vi "2D_template.vi"() -> ()   [LabVIEW 2014]
uses:
  support/Message Queue/Kapitza Message Queue.lvlib
  support/User Event - Stop/Kapitza User Event - Stop.lvlib
  support/Message Queue/Enqueue Message (Single).vi
  Classes/2D/IV/IV.lvclass
  Classes/2D/IV/data/IV_data.lvclass
  Classes/2D/IV/meas/IV_meas.lvclass
panel:
  in  "Additional Options_enum":enum32{"Page 1", "Page 2"}(tab)
  in  "Additional options":bool
  in  "Graphs":enum32{"IV", "dV/dI (I)"}(tab)
  out "IV":cluster{"X":dbl[], "Y":dbl[]}[](graph)
  out "dV/dI (I)":cluster{"X":dbl[], "Y":dbl[]}[](graph) caption="IV"
  out "Current Step":dbl
  out "dV/dI":dbl caption="dV/dI, Ohm"
  in  "File Path Control":path=path "C:/Users/Sergei/Documents"
  in  "Driver 1":path=path "C:/Users/Sergei/YandexDisk/Лаборатория/Projects/Kapitza_prealpha/Drivers/Simulator.vi" caption="Current source driver"
  in  "Driver 2":path=path "C:/Users/Sergei/YandexDisk/Лаборатория/Projects/Kapitza_prealpha/Drivers/Simulator.vi" caption="Voltmeter driver"
  in  "Address 2":refnum<visa-resource-name> caption="Voltmeter"
  in  "Address 1":refnum<visa-resource-name> caption="Current source"
  in  "Stop":bool
  in  "Sample Name":string
  in  "Max":dbl caption="Max current, uA"
  in  "Step":dbl caption="Current step, uA"
  in  "Init":dbl caption="Init current, uA"
  in  "x0,5 step":bool
  out "V":dbl caption="V, uV"
  out "I":dbl caption="I, uA"
  in  "x2 step":bool
  in  "Start":bool
  # "uA"
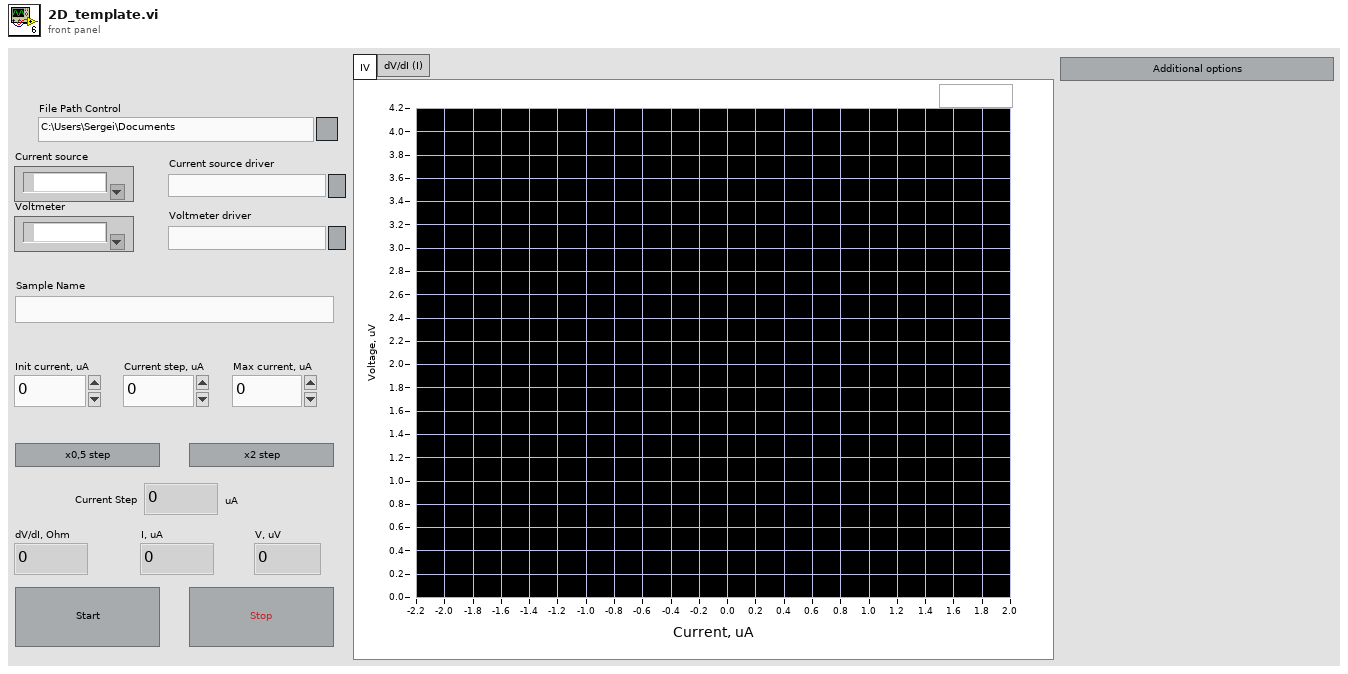
[diagram p1: front panel]
types:
  T1 = typedef "Kapitza Message Queue.lvlib/All Message Queues.ctl" = cluster{"UI":refnum<queue>}
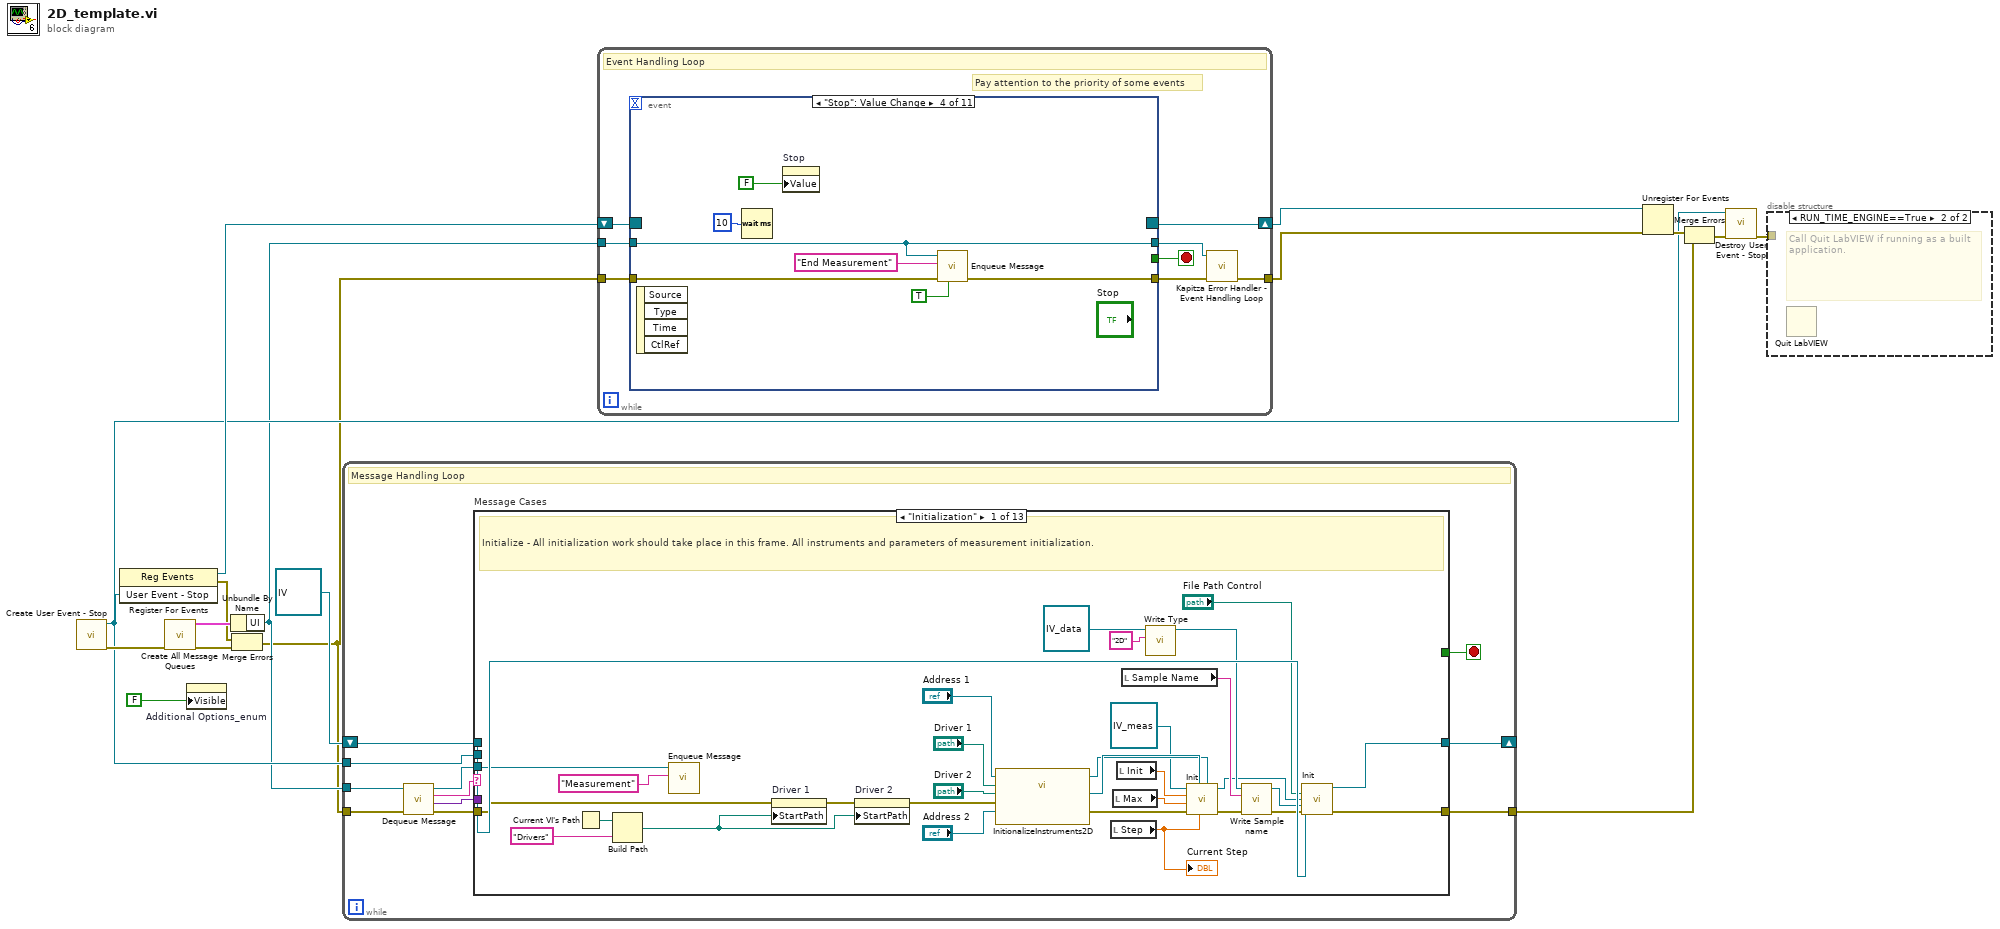
[diagram p0: block diagram]
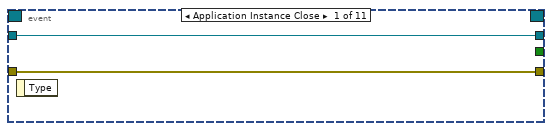
[diagram p3: hidden frame]
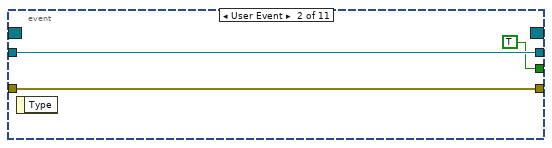
[diagram p4: hidden frame]
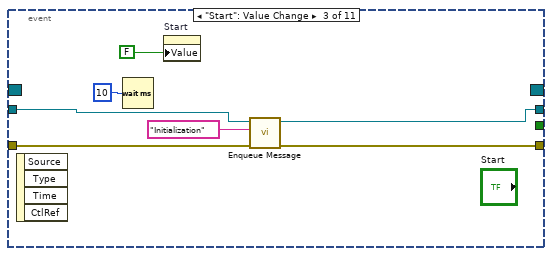
[diagram p5: hidden frame]
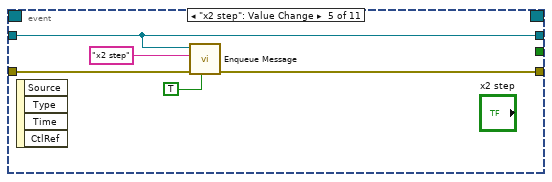
[diagram p6: hidden frame]
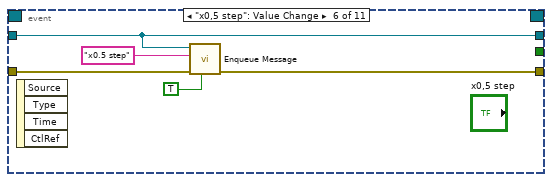
[diagram p7: hidden frame]
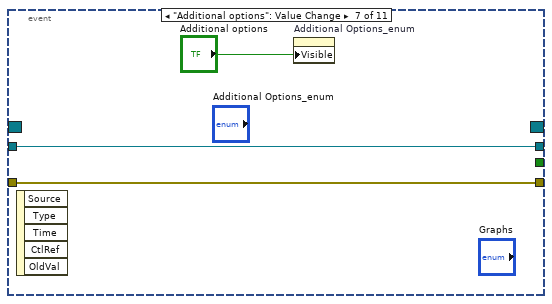
[diagram p8: hidden frame]
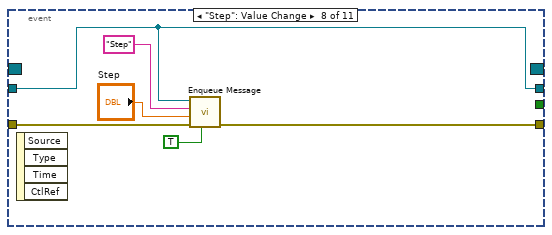
[diagram p9: hidden frame]
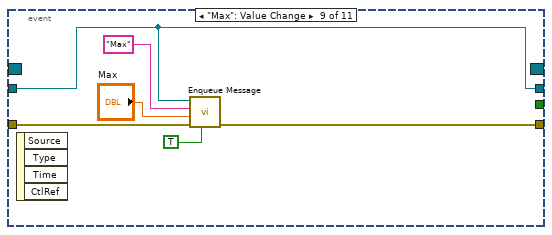
[diagram p10: hidden frame]
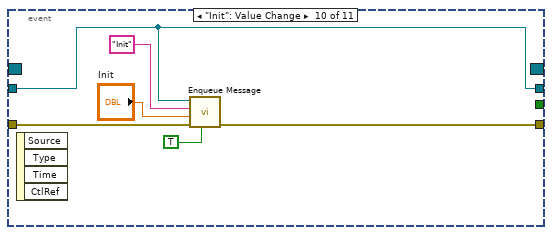
[diagram p11: hidden frame]
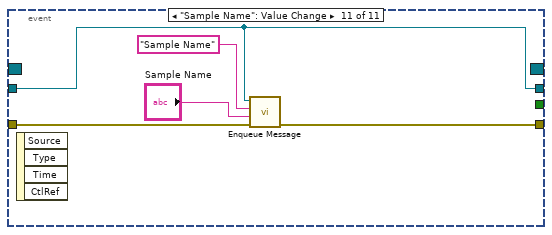
[diagram p12: hidden frame]
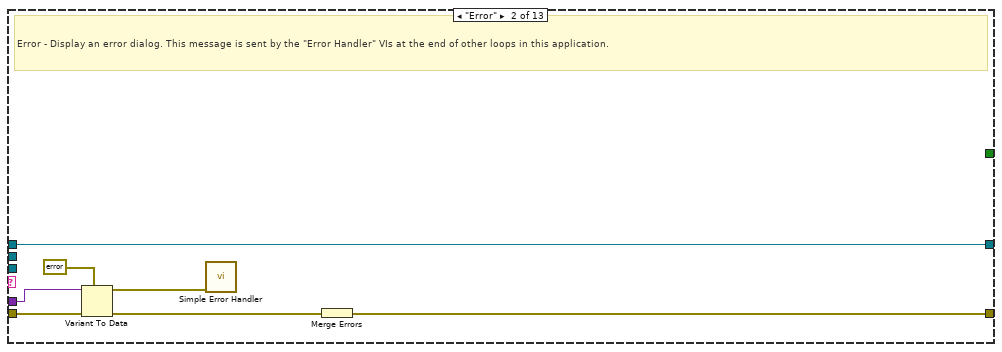
[diagram p13: hidden frame]
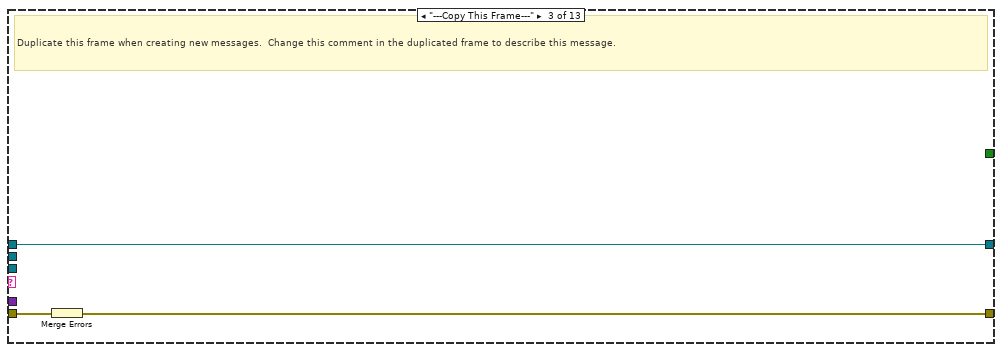
[diagram p14: hidden frame]
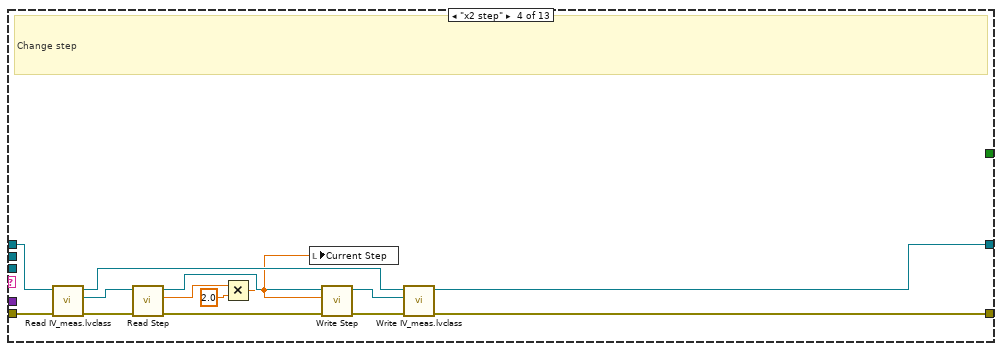
[diagram p15: hidden frame]
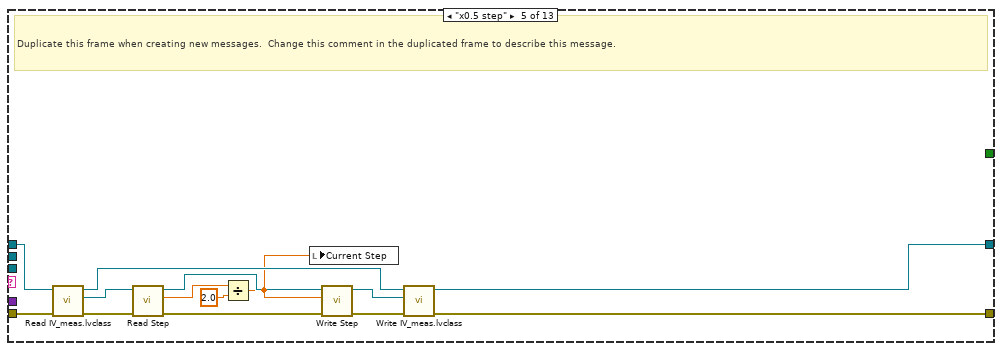
[diagram p16: hidden frame]
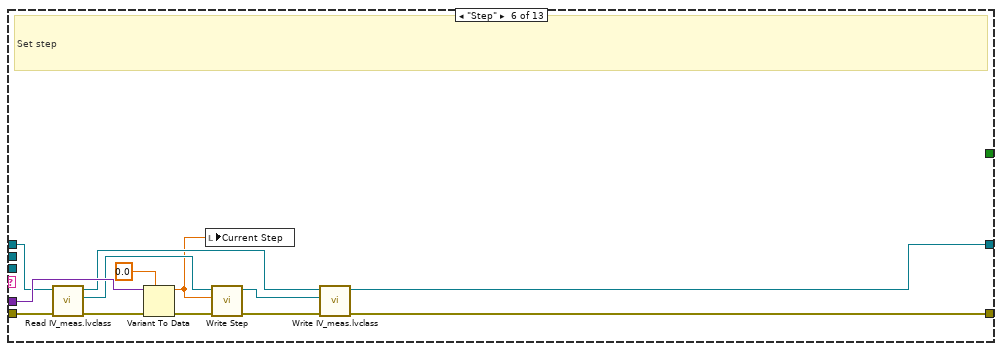
[diagram p17: hidden frame]
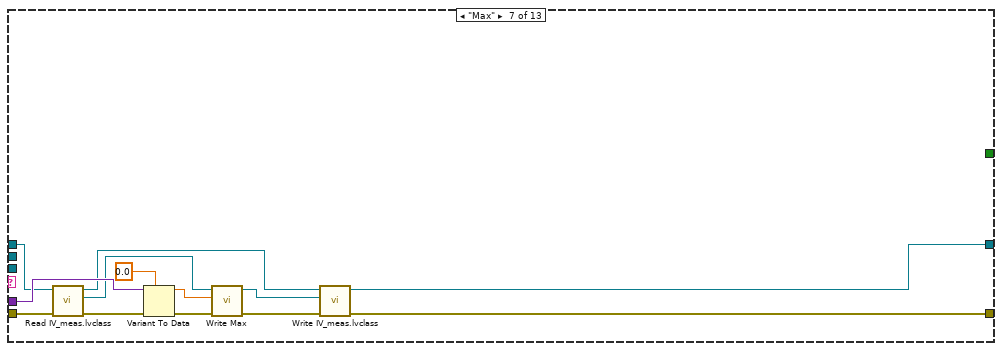
[diagram p18: hidden frame]
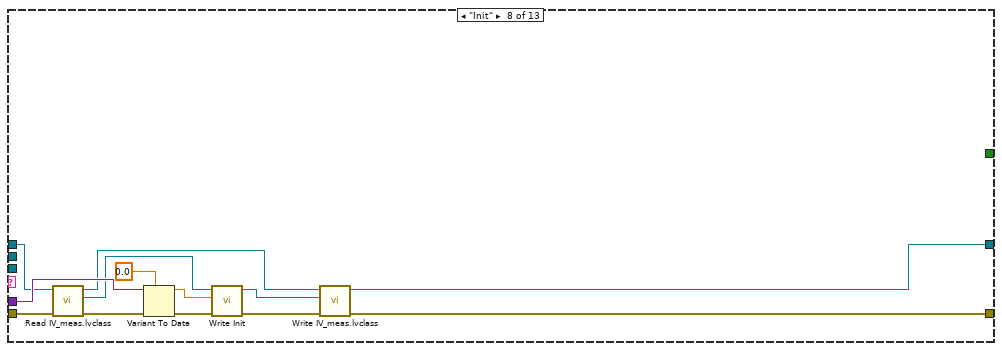
[diagram p19: hidden frame]
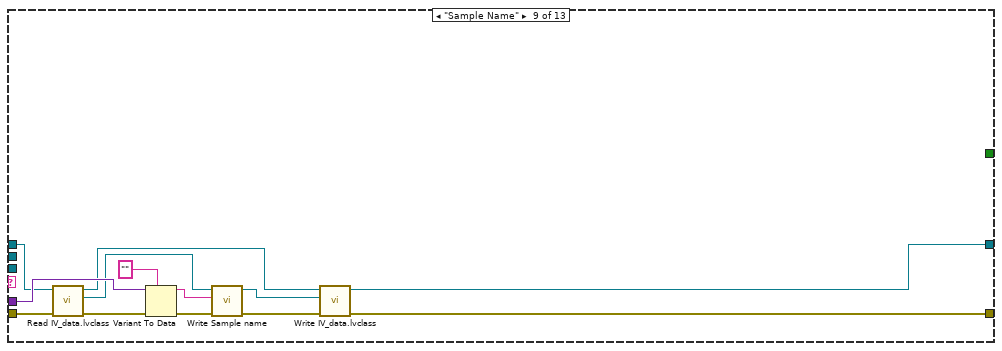
[diagram p20: hidden frame]
diagram:
  n1 = call "Create User Event - Stop.vi"() -> ("error out"=w14:errorcluster, "User Event - Stop"=w7:refnum<user-event>)  [unwired: 10 in]
  n2 = register-events(w7) -> (reference out=w8:refnum<event-registration>, error out=w6:errorcluster)  [unwired: 2 in]
  n3 = call "Create All Message Queues.vi"("error in (no error)"=w14) -> ("error out"=w4:errorcluster, "Message Queues out"=w16:T1)  [unwired: 9 in]
  n4 = property on="Additional Options_enum" class="TabCtl (strict)"("Visible"=FALSE) -> ()  [unwired: 2 in, 2 out]
  n5 = Unbundle By Name(w16) -> ("UI"=w5:refnum<queue>)
  n6 = Merge Errors(w6, w4) -> (w1:errorcluster)
  n7 = while {
    tunnel: w5 -> [w18]
    shift-right: [w26] -> _
    shift-left: refnum<class "IV.lvclass"> refnum ("IV.lvclass") -> [w27]
    tunnel: w7 -> [w24]
    tunnel: w1 -> [w23]
    tunnel: [w17] -> w15
    stop <- w25 stop-if-true
    # "Message Handling Loop"
    n8 = call "Dequeue Message.vi"("error in (no error)"=w23, "Message Queue"=w18) -> ("error out"=w22:errorcluster, "Message Data"=w20:variant, "Message"=w21:string, "dup Message Queue"=w19:refnum<queue>)  [unwired: 6 in]
    n9 = case "Message Cases" shown="\"Initialization\"" w21 {
      tunnel: w19 -> [w40 _ _ _ _ _ _ _ _ w158 w183 w195 _]
      tunnel: w22 -> [w45 w65 w68 w76 w84 w101 w115 w129 w141 w157 w177 w188 w196]
      tunnel: [w29 w59 w66 w75 w85 w103 w111 w131 w140 w155 w182 w191 w196] -> w17
      tunnel: w27 -> [w58 w64 w67 w77 w87 w107 w120 w130 w146 w159 w184 w194 w197]
      tunnel: [w30 w64 w67 w70 w86 w104 w110 w132 w139 w154 w170 w194 w197] -> w26
      tunnel: [_ _ _ _ _ _ _ _ _ _ _ TRUE _] -> w25
      tunnel: w20 -> [_ w63 _ _ _ w109 w122 w135 w148 _ _ w185 _]
      tunnel: w24 -> [_ _ _ _ _ _ _ _ _ _ _ w190 _]
      frame "Initialization" {
        # "Initialize - All initialization work should take place in this frame. All instruments and parameters of measurement initialization."
        n10 = Current VI's Path() -> (path=w47:path)
        n11 = Build Path(base path=w47, name or relative path="Drivers") -> (appended path=w43:path)
        n12 = call-poly "Enqueue Message.vi"("Message"="Measurement", "Message Queue"=w40) -> ()  [unwired: 8 in, 2 out]
        n13 = property on="Driver 1" class="Path"(error in=w45, "StartPath"=w43) -> (error out=w44:errorcluster)  [unwired: 1 in, 1 out]
        n14 = property on="Driver 2" class="Path"(error in=w44, "StartPath"=w43) -> (error out=w42:errorcluster)  [unwired: 1 in, 1 out]
        n15 = call "InitionalizeInstruments2D.vi"("Address in"="Address 2", "error in (no error)"=w42, "Driver in"="Driver 2", "Driver 1"="Driver 1", "VISA Refnum in"="Address 1") -> ("error out"=w50:errorcluster, "Instrument out 2"=w53:refnum<class "Instrument.lvclass">, "Instrument out"=w52:refnum<class "Instrument.lvclass">)  [unwired: 4 in]
        n16 = local read "Step"() -> (w28:dbl)
        "Current Step" <- w28
        n17 = local read "Max"() -> (w31:dbl)
        n18 = local read "Init"() -> (w32:dbl)
        n19 = local read "Sample Name"() -> (w51:string)
        n20 = call "Write Type.vi"("Type"="2D", "IV_data in"=refnum<class "IV_data.lvclass"> refnum ("IV_data.lvclass")) -> ("IV_data out"=w38:refnum<class "IV_data.lvclass">)  [unwired: 8 in, 1 out]
        n21 = call-dynamic "Init.vi"("Instrument.lvclass 2"=w52, "Step"=w28, "Instrument.lvclass"=w53, "error in (no error)"=w50, "Max"=w31, "Init"=w32, "Measurement1D in"=refnum<class "IV_meas.lvclass"> refnum ("IV_meas.lvclass")) -> ("error out"=w49:errorcluster, "Measurement1D out"=w34:refnum<class "IV_meas.lvclass">)  [unwired: 3 in]
        n22 = call "Write Sample name.vi"("error in (no error)"=w49, "Sample name"=w51, "IV_data in"=w38) -> ("error out"=w48:errorcluster, "IV_data out"=w33:refnum<class "IV_data.lvclass">)  [unwired: 7 in]
        n23 = call-dynamic "Init.vi"("IV in"=w58, "Path"="File Path Control", "IV_meas.lvclass"=w34, "IV_data.lvclass"=w33, "error in (no error)"=w48) -> ("IV out"=w30:refnum<class "IV.lvclass">, "error out"=w29:errorcluster)  [unwired: 9 in]
      }
      frame "Error" {
        # "Error - Display an error dialog. This message is sent by the \"Error Handler\" VIs at the end of other loops in this application."
        n24 = Variant To Data(error in=w65, type=errorcluster {"status"=FALSE, "code"=0, "source"=""} ("error constant"), Variant=w63) -> (data=w61:errorcluster, error out=w60:errorcluster)
        n25 = call <vilib>:"Simple Error Handler.vi"("error in (no error)"=w61) -> ()  [unwired: 4 in, 5 out]
        n26 = Merge Errors(w60) -> (w59:errorcluster)
      }
      frame "---Copy This Frame---" {
        # "Duplicate this frame when creating new messages.  Change this comment in the duplicated frame to describe this message."
        n27 = Merge Errors(w68) -> (w66:errorcluster)
      }
      frame "x2 step" {
        # "Change step"
        n28 = call "Read IV_meas.lvclass.vi"("error in (no error)"=w76, "IV in"=w77) -> ("error out"=w74:errorcluster, "IV_meas.lvclass"=w79:refnum<class "IV_meas.lvclass">, "IV out"=w71:refnum<class "IV.lvclass">)  [unwired: 7 in]
        n29 = call "Read Step.vi"("error in (no error)"=w74, "IV_meas in"=w79) -> ("error out"=w73:errorcluster, "Step"=w81:dbl, "IV_meas out"=w80:refnum<class "IV_meas.lvclass">)  [unwired: 7 in]
        n30 = Multiply(x=w81, y=2.0) -> (x*y=w69:dbl)
        n31 = local write "Current Step"(w69) -> ()
        n32 = call "Write Step.vi"("error in (no error)"=w73, "Step"=w69, "IV_meas in"=w80) -> ("error out"=w72:errorcluster, "IV_meas out"=w78:refnum<class "IV_meas.lvclass">)  [unwired: 7 in]
        n33 = call "Write IV_meas.lvclass.vi"("error in (no error)"=w72, "IV_meas.lvclass"=w78, "IV in"=w71) -> ("error out"=w75:errorcluster, "IV out"=w70:refnum<class "IV.lvclass">)  [unwired: 7 in]
      }
      frame "x0.5 step" {
        # "Duplicate this frame when creating new messages.  Change this comment in the duplicated frame to describe this message."
        n34 = call "Read IV_meas.lvclass.vi"("error in (no error)"=w84, "IV in"=w87) -> ("error out"=w91:errorcluster, "IV_meas.lvclass"=w93:refnum<class "IV_meas.lvclass">, "IV out"=w88:refnum<class "IV.lvclass">)  [unwired: 7 in]
        n35 = call "Read Step.vi"("error in (no error)"=w91, "IV_meas in"=w93) -> ("error out"=w90:errorcluster, "Step"=w95:dbl, "IV_meas out"=w94:refnum<class "IV_meas.lvclass">)  [unwired: 7 in]
        n36 = Divide(x=w95, y=2.0) -> (x/y=w83:dbl)
        n37 = local write "Current Step"(w83) -> ()
        n38 = call "Write Step.vi"("error in (no error)"=w90, "Step"=w83, "IV_meas in"=w94) -> ("error out"=w89:errorcluster, "IV_meas out"=w92:refnum<class "IV_meas.lvclass">)  [unwired: 7 in]
        n39 = call "Write IV_meas.lvclass.vi"("error in (no error)"=w89, "IV_meas.lvclass"=w92, "IV in"=w88) -> ("error out"=w85:errorcluster, "IV out"=w86:refnum<class "IV.lvclass">)  [unwired: 7 in]
      }
      frame "Step" {
        # "Set step"
        n40 = call "Read IV_meas.lvclass.vi"("error in (no error)"=w101, "IV in"=w107) -> ("error out"=w99:errorcluster, "IV_meas.lvclass"=w106:refnum<class "IV_meas.lvclass">, "IV out"=w98:refnum<class "IV.lvclass">)  [unwired: 7 in]
        n41 = Variant To Data(error in=w99, type=0.0, Variant=w109) -> (data=w97:dbl, error out=w100:errorcluster)
        n42 = local write "Current Step"(w97) -> ()
        n43 = call "Write Step.vi"("error in (no error)"=w100, "Step"=w97, "IV_meas in"=w106) -> ("error out"=w102:errorcluster, "IV_meas out"=w105:refnum<class "IV_meas.lvclass">)  [unwired: 7 in]
        n44 = call "Write IV_meas.lvclass.vi"("error in (no error)"=w102, "IV_meas.lvclass"=w105, "IV in"=w98) -> ("error out"=w103:errorcluster, "IV out"=w104:refnum<class "IV.lvclass">)  [unwired: 7 in]
      }
      frame "Max" {
        n45 = call "Read IV_meas.lvclass.vi"("error in (no error)"=w115, "IV in"=w120) -> ("error out"=w114:errorcluster, "IV_meas.lvclass"=w118:refnum<class "IV_meas.lvclass">, "IV out"=w119:refnum<class "IV.lvclass">)  [unwired: 7 in]
        n46 = Variant To Data(error in=w114, type=0.0, Variant=w122) -> (data=w117:dbl, error out=w113:errorcluster)
        n47 = call "Write Max.vi"("error in (no error)"=w113, "Max"=w117, "IV_meas in"=w118) -> ("error out"=w112:errorcluster, "IV_meas out"=w116:refnum<class "IV_meas.lvclass">)  [unwired: 7 in]
        n48 = call "Write IV_meas.lvclass.vi"("error in (no error)"=w112, "IV_meas.lvclass"=w116, "IV in"=w119) -> ("error out"=w111:errorcluster, "IV out"=w110:refnum<class "IV.lvclass">)  [unwired: 7 in]
      }
      frame "Init" {
        n49 = call "Read IV_meas.lvclass.vi"("error in (no error)"=w129, "IV in"=w130) -> ("error out"=w128:errorcluster, "IV_meas.lvclass"=w126:refnum<class "IV_meas.lvclass">, "IV out"=w127:refnum<class "IV.lvclass">)  [unwired: 7 in]
        n50 = Variant To Data(error in=w128, type=0.0, Variant=w135) -> (data=w133:dbl, error out=w125:errorcluster)
        n51 = call "Write Init.vi"("error in (no error)"=w125, "Init"=w133, "IV_meas in"=w126) -> ("error out"=w123:errorcluster, "IV_meas out"=w124:refnum<class "IV_meas.lvclass">)  [unwired: 7 in]
        n52 = call "Write IV_meas.lvclass.vi"("error in (no error)"=w123, "IV_meas.lvclass"=w124, "IV in"=w127) -> ("error out"=w131:errorcluster, "IV out"=w132:refnum<class "IV.lvclass">)  [unwired: 7 in]
      }
      frame "Sample Name" {
        n53 = call "Read IV_data.lvclass.vi"("error in (no error)"=w141, "IV in"=w146) -> ("error out"=w138:errorcluster, "IV_data.lvclass"=w145:refnum<class "IV_data.lvclass">, "IV out"=w142:refnum<class "IV.lvclass">)  [unwired: 7 in]
        n54 = Variant To Data(error in=w138, type="", Variant=w148) -> (data=w144:string, error out=w137:errorcluster)
        n55 = call "Write Sample name.vi"("error in (no error)"=w137, "Sample name"=w144, "IV_data in"=w145) -> ("error out"=w136:errorcluster, "IV_data out"=w143:refnum<class "IV_data.lvclass">)  [unwired: 7 in]
        n56 = call "Write IV_data.lvclass.vi"("error in (no error)"=w136, "IV_data.lvclass"=w143, "IV in"=w142) -> ("error out"=w140:errorcluster, "IV out"=w139:refnum<class "IV.lvclass">)  [unwired: 7 in]
      }
      frame "End Measurement" {
        # "End of the measurement contains three parts:  actions need to be provided to off instruments correctly, creation of results and saving them"
        n57 = Flush Queue(queue=w158, error in (no error)=w157) -> (error out=w156:errorcluster)  [unwired: 2 out]
        n58 = call-dynamic "End.vi"("error in (no error)"=w156, "IV in"=w159) -> ("error out"=w152:errorcluster, "IV out"=w153:refnum<class "IV.lvclass">)  [unwired: 8 in]
        n59 = call "Create Result.vi"("error in (no error)"=w152, "IV in"=w153) -> ("error out"=w149:errorcluster, "Text"=w150:string, "IV out"=w151:refnum<class "IV.lvclass">)  [unwired: 7 in]
        n60 = call-dynamic "Save.vi"("error in (no error)"=w149, "Text"=w150, "IV in"=w151) -> ("error out"=w155:errorcluster, "IV out"=w154:refnum<class "IV.lvclass">)  [unwired: 7 in]
      }
      frame "Measurement" {
        # "Main measurement frame. This frame repeats until reach end condition. Here also all graphs are drawn."
        n61 = call-dynamic "Measurement.vi"("error in (no error)"=w177, "IV in"=w184) -> ("error out"=w164:errorcluster, "IV out"=w169:refnum<class "IV.lvclass">)  [unwired: 6 in, 2 out]
        n62 = Wait (ms)(milliseconds to wait=u32 100) -> ()  [unwired: 1 out]
        n63 = call "Get Graph.vi"("error in (no error)"=w164, "IV in"=w169) -> ("error out"=w163:errorcluster, "Y"=w165:dbl[], "X"=w167:dbl[], "IV out"=w168:refnum<class "IV.lvclass">, "dY/dX"=w166:dbl[])  [unwired: 5 in]
        n64 = call "Convert to Dynamic Data4"("Array"=w167) -> ("Dynamic Data Type"=w172:dynamicdata)  [unwired: 3 in]
        n65 = call "Convert to Dynamic Data3"("Array"=w166) -> ("Dynamic Data Type"=w173:dynamicdata)  [unwired: 3 in]
        n66 = call "Convert to Dynamic Data"("Array"=w167) -> ("Dynamic Data Type"=w175:dynamicdata)  [unwired: 3 in]
        n67 = call "Convert to Dynamic Data2"("Array"=w165) -> ("Dynamic Data Type"=w180:dynamicdata)  [unwired: 3 in]
        n68 = call-dynamic "Get point.vi"("error in (no error)"=w163, "IV in"=w168) -> ("error out"=w178:errorcluster, "y"=w161:dbl, "x"=w162:dbl, "IV out"=w170:refnum<class "IV.lvclass">)  [unwired: 6 in]
        "I" <- w162
        "V" <- w161
        n69 = call "Build XY Graph2"("Y Input"=w173, "X Input"=w172) -> ("XY Graph"=→"dV/dI (I)":cluster{"X":dbl[], "Y":dbl[]}[])  [unwired: 8 in, 1 out]
        n70 = call "Build XY Graph"("error in (no error)"=w178, "Y Input"=w180, "X Input"=w175) -> ("error out"=w176:errorcluster, "XY Graph"=→"IV":cluster{"X":dbl[], "Y":dbl[]}[])  [unwired: 7 in]
        n71 = Divide(x=w161, y=w162) -> (x/y=→"dV/dI":dbl)
        n72 = call-poly "Enqueue Message.vi"("error in (no error)"=w176, "Message"="Measurement", "Message Queue"=w183) -> ("error out"=w182:errorcluster)  [unwired: 7 in, 1 out]
      }
      frame "Exit" {
        # "Exit - Exit the application."
        n73 = Release Queue(queue=w195, error in (no error)=w188) -> (error out=w192:errorcluster)  [unwired: 1 in, 2 out]
        n74 = call "Fire User Event - Stop.vi"("User Event - Stop"=w190) -> ("error out"=w189:errorcluster)  [unwired: 10 in]
        n75 = Variant To Data(type=errorcluster {"status"=FALSE, "code"=0, "source"=""} ("error constant"), Variant=w185) -> (data=w186:errorcluster)  [unwired: 1 in, 1 out]
        n76 = Merge Errors(w189, w192) -> (w191:errorcluster)
        n77 = call <vilib>:"Simple Error Handler.vi"("error in (no error)"=w186) -> ()  [unwired: 4 in, 5 out]
      }
      frame Default {
        # "'Default' case only runs if there is a message that isn't defined in any of the other cases"
      }
    }
  }
  n78 = while {
    tunnel: w5 -> [w205]
    shift-right: [w203] -> w11
    shift-left: w8 -> [w204]
    tunnel: [w200] -> w9
    tunnel: w1 -> [w198]
    stop <- w202 stop-if-true
    # "Pay attention to the priority of some events"
    # "Event Handling Loop"
    n79 = event shown="[3] \"Stop\": Value Change" {
      selector: w204 -> [_ _ _ _ _ _ _ _ _ _ _]
      dyn-events: [_ _ _ _ _ _ _ _ _ _ _] -> w203
      timeout: _ -> [_ _ _ _ _ _ _ _ _ _ _]
      tunnel: [_ TRUE ("Discard?") _ _ _ _ _ _ _ _ _] -> w202
      tunnel: w205 -> [w207 w210 w217 w224 w229 w232 w237 w242 w247 w253 w259]
      tunnel: [w207 w210 w216 w224 w229 w232 w237 w242 w247 w253 w259] -> w201
      tunnel: [w206 w208 w211 w218 w225 w230 w235 w238 w244 w250 w256] -> w199
      tunnel: w198 -> [w206 w208 w212 w219 w226 w231 w235 w239 w245 w251 w257]
      event Application Instance Close {
        n80 = event-data() -> ()  [unwired: 1 in, 1 out]
      }
      event User Event {
        n81 = event-data() -> ()  [unwired: 1 in, 1 out]
      }
      event "Start": Value Change {
        n82 = event-data() -> ()  [unwired: 1 in, 4 out]
        n83 = Wait (ms)(milliseconds to wait=u32 10) -> ()  [unwired: 1 out]
        n84 = property on="Start" class="Bool (strict)"("Value"=FALSE ("Start")) -> ()  [unwired: 2 in, 2 out]
        n85 = call-poly "Enqueue Message.vi"("error in (no error)"=w212, "Message"="Initialization", "Message Queue"=w217) -> ("error out"=w211:errorcluster, "dup Message Queue"=w216:refnum<queue>)  [unwired: 7 in]
      }
      event "Stop": Value Change {
        n86 = event-data() -> ()  [unwired: 1 in, 4 out]
        n87 = Wait (ms)(milliseconds to wait=u32 10) -> ()  [unwired: 1 out]
        n88 = property on="Stop" class="Bool (strict)"("Value"=FALSE ("Stop")) -> ()  [unwired: 2 in, 2 out]
        n89 = call-poly "Enqueue Message.vi"("Priority Message? (F)"=TRUE, "error in (no error)"=w219, "Message"="End Measurement", "Message Queue"=w224) -> ("error out"=w218:errorcluster)  [unwired: 6 in, 1 out]
      }
      event "x2 step": Value Change {
        n90 = event-data() -> ()  [unwired: 1 in, 4 out]
        n91 = call-poly "Enqueue Message.vi"("Priority Message? (F)"=TRUE, "error in (no error)"=w226, "Message"="x2 step", "Message Queue"=w229) -> ("error out"=w225:errorcluster)  [unwired: 6 in, 1 out]
      }
      event "x0,5 step": Value Change {
        n92 = event-data() -> ()  [unwired: 1 in, 4 out]
        n93 = call-poly "Enqueue Message.vi"("Priority Message? (F)"=TRUE, "error in (no error)"=w231, "Message"="x0.5 step", "Message Queue"=w232) -> ("error out"=w230:errorcluster)  [unwired: 6 in, 1 out]
      }
      event "Additional options": Value Change {
        n94 = event-data() -> ()  [unwired: 1 in, 5 out]
        n95 = property on="Additional Options_enum" class="TabCtl (strict)"("Visible"="Additional options") -> ()  [unwired: 2 in, 2 out]
      }
      event "Step": Value Change {
        n96 = event-data() -> ()  [unwired: 1 in, 4 out]
        n97 = call-poly "Enqueue Message.vi"("Priority Message? (F)"=TRUE, "error in (no error)"=w239, "Message Data"="Step", "Message"="Step", "Message Queue"=w242) -> ("error out"=w238:errorcluster)  [unwired: 5 in, 1 out]
      }
      event "Max": Value Change {
        n98 = event-data() -> ()  [unwired: 1 in, 4 out]
        n99 = call-poly "Enqueue Message.vi"("Priority Message? (F)"=TRUE, "error in (no error)"=w245, "Message Data"="Max", "Message"="Max", "Message Queue"=w247) -> ("error out"=w244:errorcluster)  [unwired: 5 in, 1 out]
      }
      event "Init": Value Change {
        n100 = event-data() -> ()  [unwired: 1 in, 4 out]
        n101 = call-poly "Enqueue Message.vi"("Priority Message? (F)"=TRUE, "error in (no error)"=w251, "Message Data"="Init", "Message"="Init", "Message Queue"=w253) -> ("error out"=w250:errorcluster)  [unwired: 5 in, 1 out]
      }
      event "Sample Name": Value Change {
        n102 = event-data() -> ()  [unwired: 1 in, 4 out]
        n103 = call-poly "Enqueue Message.vi"("error in (no error)"=w257, "Message Data"="Sample Name", "Message"="Sample Name", "Message Queue"=w259) -> ("error out"=w256:errorcluster)  [unwired: 6 in, 1 out]
      }
    }
    n104 = call "Kapitza Error Handler - Event Handling Loop.vi"("error in (no error)"=w199, "Message Queue"=w201) -> ("dup error in"=w200:errorcluster)  [unwired: 8 in, 1 out]
  }
  n105 = Unregister For Events(event registration refnum=w11, error in=w9) -> (error out=w12:errorcluster)
  n106 = Merge Errors(w12, w15) -> (w13:errorcluster)
  n107 = call "Destroy User Event - Stop.vi"("error in (no error)"=w13, "User Event - Stop"=w7) -> ("error out"=w10:errorcluster)  [unwired: 9 in]
  n108 = disable-structure shown="RUN_TIME_ENGINE==True" {
    disable-tunnel: w10 -> [_ _]
    frame condition #0 (active) {
    }
    frame condition #1 {
      # "Call Quit LabVIEW if running as a built application."
      n109 = Quit LabVIEW() -> ()  [unwired: 1 in]
    }
  }
